vi "ECAT Close FoE Write.vi"(8 "Error In":errorcluster, 11 "Slave Ref in":refnum<k21>) -> (0 "Error Out":errorcluster, 3 "Slave Ref out":refnum<k21>)   [LabVIEW 2016, in "Scan Engine Custom Device.lvlib"]
uses:
  Scan Engine Custom Device.lvlib
  <resource>/objmgr/IndComECAT.rc
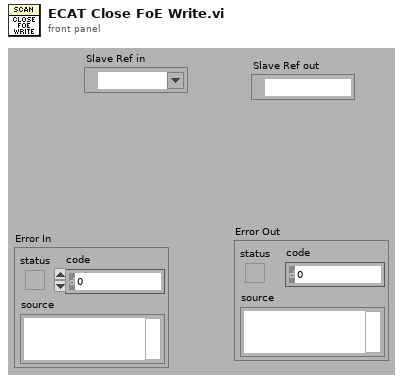
[diagram p1: front panel]
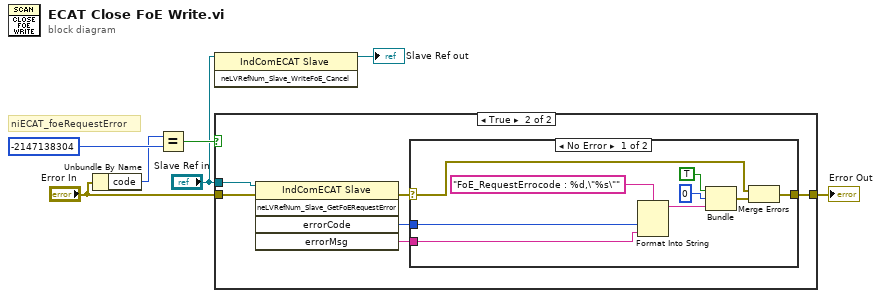
[diagram p0: block diagram]
diagram:
  # "niECAT_foeRequestError"
  n1 = Unbundle By Name("Error In") -> ("code"=w4:i32)
  n2 = Equal?(x=w4, y=-2147138304) -> (x = y?=w7:bool)
  n3 = invoke class="IndComECAT Slave" method="neLVRefNum_Slave_WriteFoE_Cancel"(reference="Slave Ref in") -> (reference out=→"Slave Ref out":refnum<k21>)  [unwired: 2 in, 2 out]
  n4 = case shown="True" w7 {
    tunnel: "Error In" -> [w8 w12]
    tunnel: [w8 w10] -> w3
    tunnel: "Slave Ref in" -> [_ w9]
    frame False {
    }
    frame True {
      n5 = invoke class="IndComECAT Slave" method="neLVRefNum_Slave_GetFoERequestError"(reference=w9, error in=w12) -> (error out=w14:errorcluster, "errorCode"=w13:u32, "errorMsg"=w11:string)  [unwired: 3 in, 2 out]
      n6 = case shown="No Error" w14 {
        selector: w14 -> [w15 w24]
        tunnel: [w18 w24] -> w10
        tunnel: w13 -> [w16 _]
        tunnel: w11 -> [w17 _]
        frame No Error {
          n7 = Format Into String(format string="FoE_RequestErrocode : %d,\"%s\"", w16, w17) -> (resulting string=w20:string)  [unwired: 2 in, 1 out]
          n8 = Bundle("status"=TRUE, "code"=0, w20) -> (w19:cluster{"status":bool, "code":i32, string})  [unwired: 1 out]
          n9 = Merge Errors(w15, w19) -> (w18:errorcluster)
        }
        frame Error {
        }
      }
    }
  }
  "Error Out" <- w3
